vi "Translate_CLUSTER.vi"(8 "error IN":errorcluster, 10 "Cle":string, 11 "Clust Refnum":refnum<vi>) -> (0 "error out":errorcluster)   [LabVIEW 2013]
uses:
  Dictionnary/EnumCommandDictionnaire.ctl
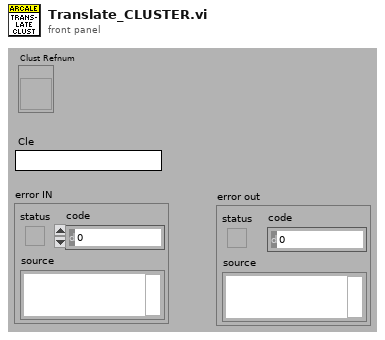
[diagram p1: front panel]
types:
  T1 = typedef "EnumCommandDictionnaire.ctl" = enum16{"Load", "Translate", "Save", "GetDico", "Set : A traduire = Vrai", "Set : A Traduire = Faux", "SetDico"}
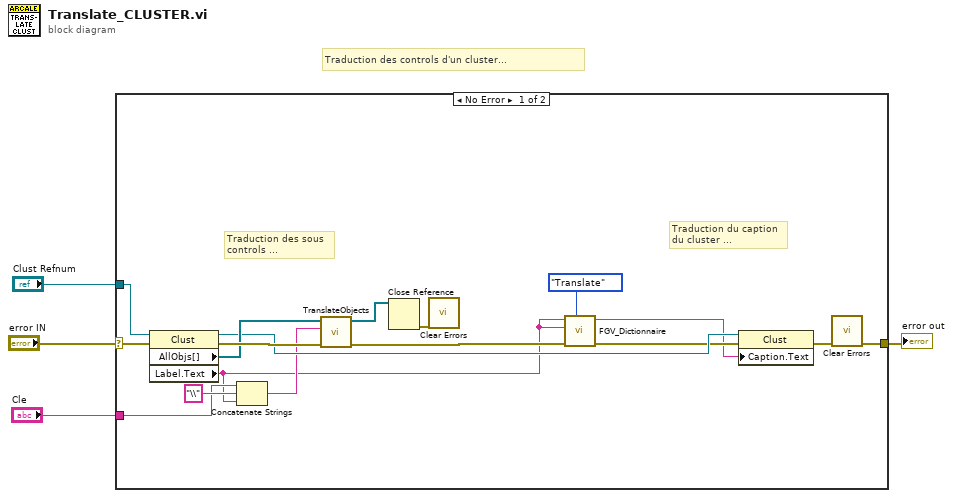
[diagram p0: block diagram]
diagram:
  # "Traduction des controls d'un cluster..."
  n1 = case shown="No Error" "error IN" {
    selector: "error IN" -> [w21 w22]
    tunnel: "Clust Refnum" -> [w20 _]
    tunnel: "Cle" -> [w8 _]
    tunnel: [w6 w22] -> w1
    frame No Error {
      # "Traduction du caption\ndu cluster ..."
      # "Traduction des sous \ncontrols ..."
      n2 = property class="Clust"(reference=w20, error in=w21) -> (reference out=w14:refnum<vi>, error out=w19:errorcluster, "AllObjs[]"=w18:refnum<vi>[], "Label.Text"=w5:string)
      n3 = Concatenate Strings(w8, "\\" ("string"), w5) -> (w13:string)
      n4 = call "TranslateObjects.vi"("errorIN"=w19, "Cle"=w13, "AllObjs[]In"=w18) -> ("error out"=w10:errorcluster, "AllObjs[]Out"=w15:refnum<vi>[])  [unwired: 7 in]
      n5 = Close Reference(reference=w15) -> (error out=w16:errorcluster)  [unwired: 1 in]
      n6 = call <vilib>:"Clear Errors.vi"("error in (no error)"=w16) -> ()  [unwired: 6 in, 1 out]
      n7 = call "FGV_Dictionnaire.vi"("Command"=EnumCommandDictionnaire."Translate", "error in (no error)"=w10, "Chaîne"=w5, "Clé"=w5) -> ("error out"=w9:errorcluster, "Traduction"=w7:string)  [unwired: 5 in, 1 out]
      n8 = property class="Clust"(reference=w14, error in=w9, "Caption.Text"=w7) -> (error out=w12:errorcluster)  [unwired: 1 out]
      n9 = call <vilib>:"Clear Errors.vi"("error in (no error)"=w12) -> ("error out"=w6:errorcluster)  [unwired: 6 in]
    }
    frame Error {
    }
  }
  "error out" <- w1
